vi "drawDXFobjs.vi"(7 "Flip in horizontal line?":bool, 11 "objs to draw":cluster{string, dbl[]}[](array[cluster])) -> (3 "picture":picture)   [LabVIEW 2016, in "Dxf.lvlib"]
uses:
  Dxf.lvlib
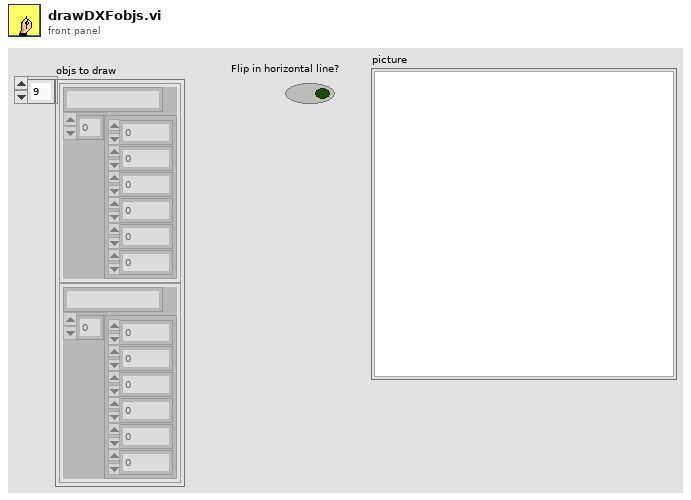
[diagram p1: front panel]
types:
  T1 = cluster{"left":i16, "top":i16, "right":i16, "bottom":i16}
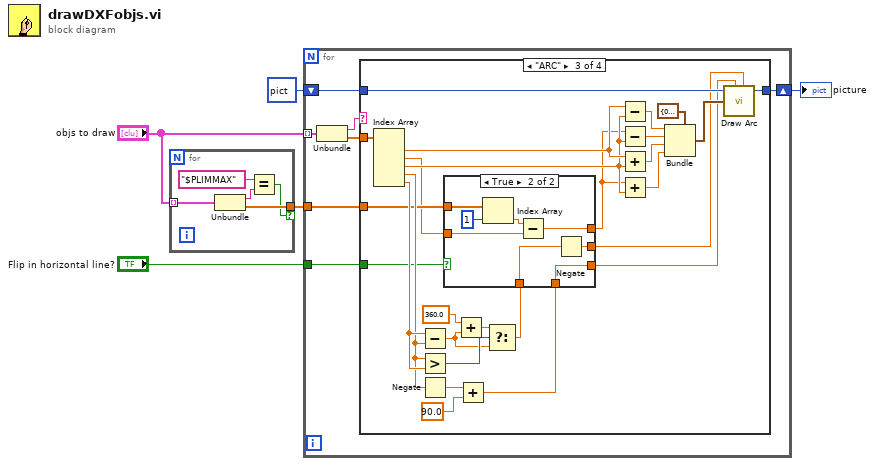
[diagram p0: block diagram]
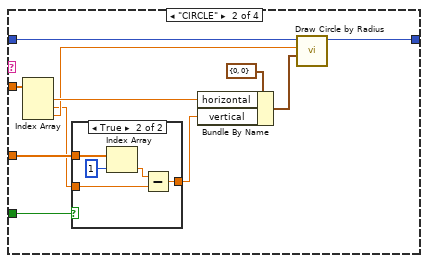
[diagram p3: hidden frame]
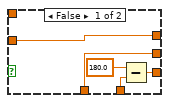
[diagram p5: hidden frame]
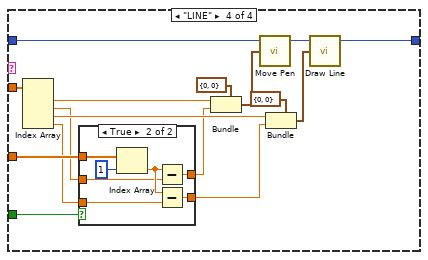
[diagram p6: hidden frame]
diagram:
  n1 = for {
    tunnel: "objs to draw" -> [w10] mode=indexing
    tunnel: [w7] -> w3 if=w6
    n2 = Unbundle(w10) -> (w9:string, w7:dbl[])
    n3 = Equal?(x="$PLIMMAX", y=w9) -> (x = y?=w6:bool)
  }
  n4 = for {
    tunnel: "objs to draw" -> [w17] mode=indexing
    shift-right: [w15] -> w1
    shift-left: picture data[5B] ("picture") -> [w16]
    tunnel: w3 -> [w12]
    tunnel: "Flip in horizontal line?" -> [w11]
    n5 = Unbundle(w17) -> (w14:string, w13:dbl[])
    n6 = case shown="\"ARC\"" w14 {
      tunnel: w16 -> [w18 w29 w48 w89]
      tunnel: [w18 w26 w61 w88] -> w15
      tunnel: w13 -> [_ w25 w62 w91]
      tunnel: w12 -> [_ w22 w51 w81]
      tunnel: w11 -> [_ w19 w39 w76]
      frame Default {
      }
      frame "CIRCLE" {
        n7 = Index Array(array=w25) -> (element #1=w24:dbl, element #2=w21:dbl, element #3=w23:dbl)  [unwired: 3 in]
        n8 = case shown="True" w19 {
          tunnel: w22 -> [_ w35]
          tunnel: w21 -> [w30 w33]
          tunnel: [w30 w31] -> w20
          frame False {
          }
          frame True {
            n9 = Index Array(array=w35, index=1) -> (element=w34:dbl)
            n10 = Subtract(x=w34, y=w33) -> (x-y=w31:dbl)
          }
        }
        n11 = Bundle By Name(cluster=cluster{"horizontal":i16, "vertical":i16} {"horizontal"=0, "vertical"=0} ("pixel center"), "horizontal"=w24, "vertical"=w20) -> (w27:cluster{"horizontal":i16, "vertical":i16})
        n12 = call <vilib>:"Draw Circle by Radius.vi"("pixel center"=w27, "radius"=w23, "picture"=w29) -> ("new picture"=w26:picture)  [unwired: 8 in]
      }
      frame "ARC" {
        n13 = Index Array(array=w62) -> (element #1=w59:dbl, element #2=w50:dbl, element #3=w56:dbl, element #4=w52:dbl, element #5=w53:dbl)  [unwired: 5 in]
        n14 = Subtract(x=w53, y=w52) -> (x-y=w42:dbl)
        n15 = Greater?(x=w52, y=w53) -> (0:w44:bool)
        n16 = Negate(x=w52) -> (-x=w41:dbl)
        n17 = Add(x=360.0, y=w42) -> (x+y=w40:dbl)
        n18 = Add(x=w41, y=90.0) -> (x+y=w38:dbl)
        n19 = Select(t=w40, s=w44, f=w42) -> (s? t:f=w45:dbl)
        n20 = case shown="True" w39 {
          tunnel: [w64 w75] -> w36
          tunnel: w51 -> [_ w74]
          tunnel: w50 -> [w63 w73]
          tunnel: [w63 w72] -> w49
          tunnel: w45 -> [w64 w69]
          tunnel: w38 -> [w66 w68]
          tunnel: [w65 w68] -> w37
          frame False {
            n21 = Subtract(x=180.0, y=w66) -> (x-y=w65:dbl)
          }
          frame True {
            n22 = Index Array(array=w74, index=1) -> (element=w70:dbl)
            n23 = Subtract(x=w70, y=w73) -> (x-y=w72:dbl)
            n24 = Negate(x=w69) -> (-x=w75:dbl)
          }
        }
        n25 = Subtract(x=w59, y=w56) -> (x-y=w58:dbl)
        n26 = Subtract(x=w49, y=w56) -> (x-y=w54:dbl)
        n27 = Add(x=w59, y=w56) -> (x+y=w57:dbl)
        n28 = Add(x=w49, y=w56) -> (x+y=w55:dbl)
        n29 = Bundle(cluster=T1 {"left"=0, "top"=0, "right"=0, "bottom"=0} ("rect"), "left"=w58, "top"=w54, "right"=w57, "bottom"=w55) -> (w47:T1)
        n30 = call <vilib>:"Draw Arc.vi"("picture"=w48, "start angle[degrees]"=w37, "rect"=w47, "arc size[degrees]"=w36) -> ("new picture"=w61:picture)  [unwired: 5 in]
      }
      frame "LINE" {
        n31 = Index Array(array=w91) -> (element #1=w83:dbl, element #2=w78:dbl, element #3=w82:dbl, element #4=w80:dbl)  [unwired: 4 in]
        n32 = case shown="True" w76 {
          tunnel: w81 -> [_ w99]
          tunnel: w80 -> [w93 w97]
          tunnel: [w93 w96] -> w79
          tunnel: w78 -> [w92 w95]
          tunnel: [w92 w94] -> w77
          frame False {
          }
          frame True {
            n33 = Index Array(array=w99, index=1) -> (element=w98:dbl)
            n34 = Subtract(x=w98, y=w95) -> (x-y=w94:dbl)
            n35 = Subtract(x=w98, y=w97) -> (x-y=w96:dbl)
          }
        }
        n36 = Bundle(cluster=cluster{"x":i16, "y":i16} {"x"=0, "y"=0} ("new position"), "x"=w83, "y"=w77) -> (w84:cluster{"x":i16, "y":i16})
        n37 = call <vilib>:"Move Pen.vi"("new position"=w84, "picture"=w89) -> ("new picture"=w90:picture)  [unwired: 3 in]
        n38 = Bundle(cluster=cluster{"x":i16, "y":i16} {"x"=0, "y"=0} ("end point"), "x"=w82, "y"=w79) -> (w85:cluster{"x":i16, "y":i16})
        n39 = call <vilib>:"Draw Line.vi"("picture"=w90, "end point"=w85) -> ("new picture"=w88:picture)  [unwired: 7 in]
      }
    }
  }
  "picture" <- w1
